vi "SignalGenerator.vi"(1 "stop (T)":bool=TRUE, 2 "Frequency":dbl=10.1, 3 "Amplitude":dbl=1.0) -> ()   [LabVIEW 2015]
panel:
  in  "error in":errorcluster
  out "error out":errorcluster
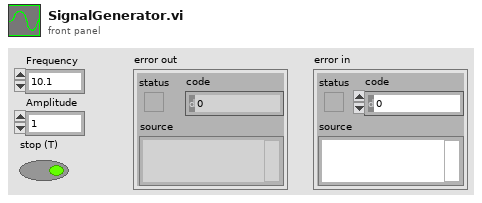
[diagram p1: front panel]
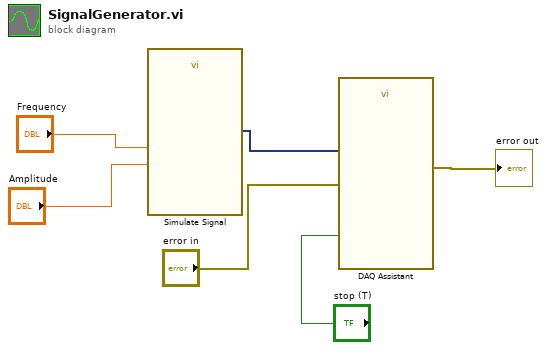
[diagram p0: block diagram]
diagram:
  n1 = call "Simulate Signal"("Frequency"="Frequency", "Amplitude"="Amplitude") -> ("Sine"=w4:dynamicdata)  [unwired: 12 in, 1 out]
  n2 = call "DAQ Assistant"("data"=w4, "error in"="error in", "stop (T)"="stop (T)") -> ("error out"=→"error out":errorcluster)  [unwired: 15 in, 1 out]
